vi "Write Config file.vi"(8 "error in (no error)":errorcluster, 10 "Config file":string, 11 "SysLogbook in":refnum<class "SysLogbook.lvclass">) -> (0 "error out":errorcluster, 3 "SysLogbook out":refnum<class "SysLogbook.lvclass">)   [LabVIEW 2014, in "SysLogbook.lvclass"]
uses:
  SysLogbook.lvclass
  SysLogbook.lvclass/SysLogbook.ctl
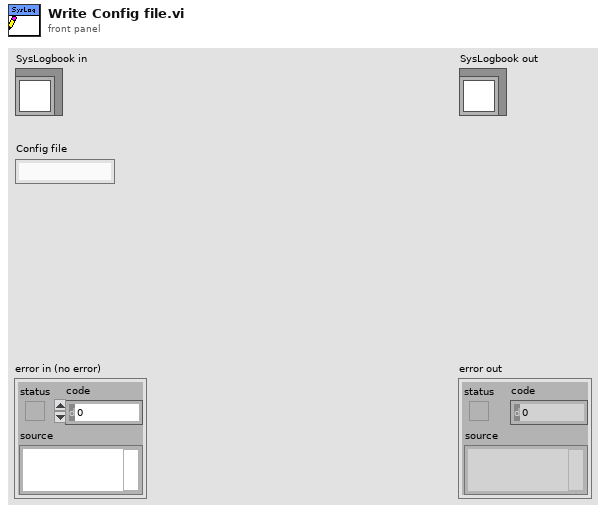
[diagram p1: front panel]
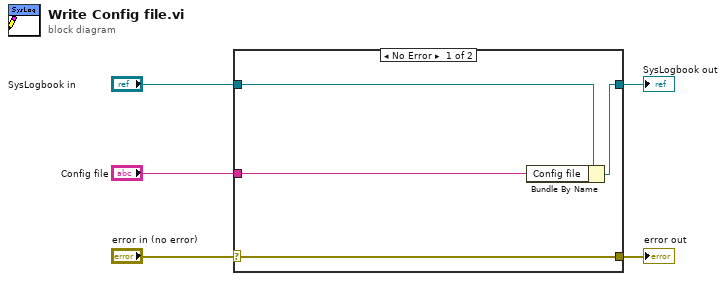
[diagram p0: block diagram]
diagram:
  n1 = case shown="No Error" "error in (no error)" {
    selector: "error in (no error)" -> [w9 w10]
    tunnel: [w9 w10] -> w4
    tunnel: [w7 w11] -> w2
    tunnel: "SysLogbook in" -> [w8 w11]
    tunnel: "Config file" -> [w6 _]
    frame No Error {
      n2 = Bundle By Name(cluster=w8, "Config file"=w6) -> (w7:refnum<class "SysLogbook.lvclass">)
    }
    frame Error {
    }
  }
  "error out" <- w4
  "SysLogbook out" <- w2
